vi "make 2d scan file.vi"() -> ()   [LabVIEW 2013]
uses:
  scan parameters.ctl
panel:
  in  "2nd as a scan":bool
  in  "start scan":i32
  in  "precision (12)":i16=12
  in  "reverse which par is scanned":bool
  in  "2D scan details":T2(array[cluster])=[{"Scan parameters"={"Scan Start"=0.00012962, "Scan End"=0.00012964, "Scan Step Size"=2e-09, "# Shots Each Step"=2, "single direction?"=TRUE}, "device and variable preamble"="Device = \"HeatHighlandT564\"\nVariable = \"Discharge timing s\""}, {"Scan parameters"={"Scan Start"=20.0, "Scan End"=50.0, "Scan Step Size"=2.0, "# Shots Each Step"=20, "single direction?"=TRUE}, "device and variable preamble"="Device = \"PL1-PresCtrl-Low1\"\nVariable = \"P. Control Down (Torr)\""}] {"Scan parameters"."Scan Start" format="%#.9p"; "Scan parameters"."Scan End" format="%#.9p"; "Scan parameters"."Scan Step Size" format="%#.9p"}
  out "spreadsheet string":string
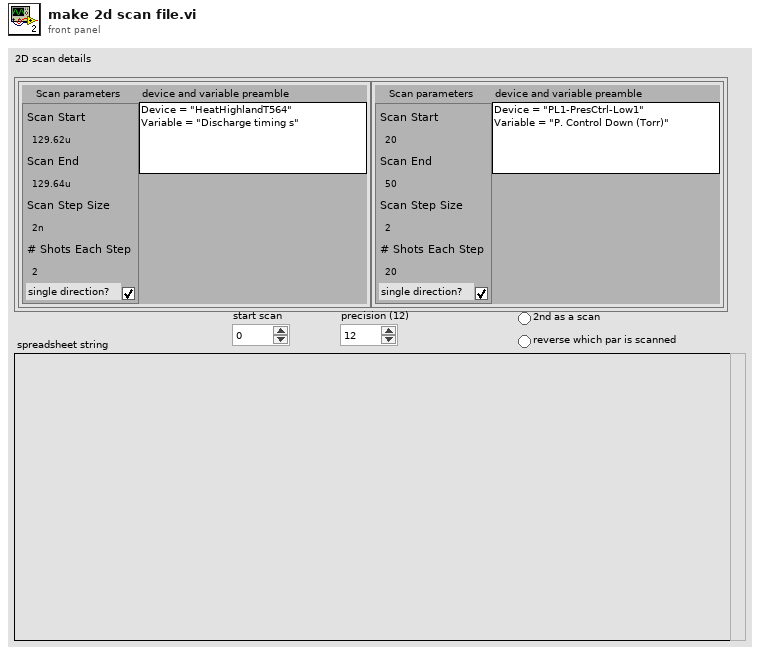
[diagram p1: front panel]
types:
  T1 = typedef "scan parameters.ctl" = cluster{"Scan Start":dbl, "Scan End":dbl, "Scan Step Size":dbl, "# Shots Each Step":u32, "single direction?":bool}
  T2 = cluster{"Scan parameters":T1, "device and variable preamble":string}[]
  T3 = cluster{"Scan parameters":T1, "device and variable preamble":string}
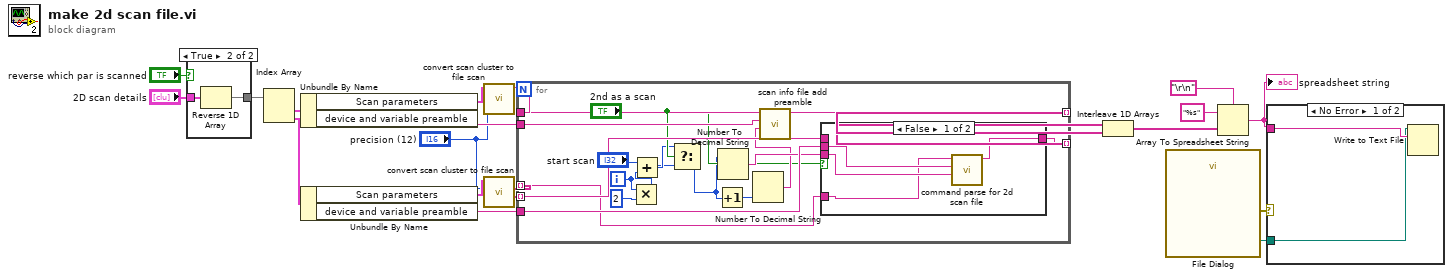
[diagram p0: block diagram]
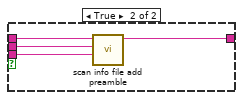
[diagram p4: hidden frame]
diagram:
  n1 = case shown="True" "reverse which par is scanned" {
    tunnel: "2D scan details" -> [w22 w24]
    tunnel: [w22 w23] -> w8
    frame False {
    }
    frame True {
      n2 = Reverse 1D Array(array=w24) -> (reversed array=w23:T2)
    }
  }
  n3 = Index Array(array=w8) -> (element #1=w6:T3, element #2=w5:T3)  [unwired: 2 in]
  n4 = Unbundle By Name(w6) -> ("Scan parameters"=w11:T1, "device and variable preamble"=w10:string)
  n5 = Unbundle By Name(w5) -> ("Scan parameters"=w4:T1, "device and variable preamble"=w3:string)
  n6 = call "convert scan cluster to file scan.vi"("precision (12)"="precision (12)", "Scan parameters"=w11) -> ("spreadsheet string"=w21:string)  [unwired: 7 in, 2 out]
  n7 = call "convert scan cluster to file scan.vi"("precision (12)"="precision (12)", "Scan parameters"=w4) -> ("values:numshots"=w17:string[], "values"=w1:string[])  [unwired: 7 in, 1 out]
  n8 = for {
    tunnel: [w39] -> w18 mode=indexing
    tunnel: w21 -> [w40]
    tunnel: w17 -> [w37] mode=indexing
    tunnel: [w36] -> w15 mode=indexing
    tunnel: w10 -> [w35]
    tunnel: w3 -> [w34]
    tunnel: w1 -> [w29] mode=indexing
    i -> [w25]
    n9 = Multiply(x=w25, y=2) -> (x*y=w31:i32)
    n10 = Add(x="start scan", y=w31) -> (x+y=w27:i32)
    n11 = Select(t=w27, s="2nd as a scan", f=w25) -> (s? t:f=w26:i32)
    n12 = Increment(x=w26) -> (x+1=w38:i32)
    n13 = Number To Decimal String(number=w26) -> (decimal integer string=w33:string)  [unwired: 1 in]
    n14 = Number To Decimal String(number=w38) -> (decimal integer string=w32:string)  [unwired: 1 in]
    n15 = call "scan info file add preamble.vi"("scan #"=w32, "device and variable stuff"=w35, "spreadsheet string"=w40) -> ("scan text for txt file"=w39:string)  [unwired: 8 in]
    n16 = case shown="False" "2nd as a scan" {
      tunnel: w37 -> [_ w49]
      tunnel: [w43 w48] -> w36
      tunnel: w34 -> [w45 w47]
      tunnel: w33 -> [w44 w46]
      tunnel: w29 -> [w42 _]
      frame False {
        n17 = call "command parse for 2d scan file.vi"("scan #"=w44, "device and variable stuff"=w45, "spreadsheet string"=w42) -> ("scan text for txt file"=w43:string)  [unwired: 8 in]
      }
      frame True {
        n18 = call "scan info file add preamble.vi"("scan #"=w46, "device and variable stuff"=w47, "spreadsheet string"=w49) -> ("scan text for txt file"=w48:string)  [unwired: 8 in]
      }
    }
  }
  n19 = Interleave 1D Arrays(w15, w18) -> (w16:string[])
  n20 = call "File Dialog"() -> ("selected path"=w12:path, "error out"=w13:errorcluster)  [unwired: 12 in, 2 out]
  n21 = Array To Spreadsheet String(delimiter (Tab)="\r\n", array=w16, 3:"%s" ("format string")) -> (spreadsheet string=w14:string)
  "spreadsheet string" <- w14
  n22 = case shown="No Error" w13 {
    tunnel: w14 -> [w51 _]
    tunnel: w12 -> [w50 _]
    frame No Error {
      n23 = Write to Text File(file (use dialog)=w50, text=w51) -> ()  [unwired: 2 in, 3 out]
    }
    frame Error {
    }
  }
